vi "Graph_range_select_slider.vi"() -> ()   [LabVIEW 2018]
panel:
  in  "X_Slider":cluster{"Slider":dbl, "Slider":dbl}(slide)={"Slider"=0.0, "Slider"=3.61890694239291} scale=3643617600.0..3643691204.0 scale format="%<%H:%M:%S\n%d/%m/%y>T"
  in  "Y_Slide":cluster{"Slider":dbl, "Slider":dbl}(slide)={"Slider"=0.0, "Slider"=6.141304347826087} scale=-0.5..2.0
  out "Graph 2":T1(graph)
  in  "Graph 1":T1(graph)=[{"Time_Stamp"=array[63091 elements], "Current_Out"=array[63091 elements]}, {"Time_Stamp"=array[63091 elements], "Current_Out"=array[63091 elements]}, {"Time_Stamp"=array[63091 elements], "Current_Out"=array[63091 elements]}, {"Time_Stamp"=array[63091 elements], "Current_Out"=array[63091 elements]}, {"Time_Stamp"=array[63091 elements], "Current_Out"=array[63091 elements]}, {"Time_Stamp"=array[63091 elements], "Current_Out"=array[63091 elements]}, {"Time_Stamp"=array[63091 elements], "Current_Out"=array[63091 elements]}]
  # "Current [uA]"
  # "Time"
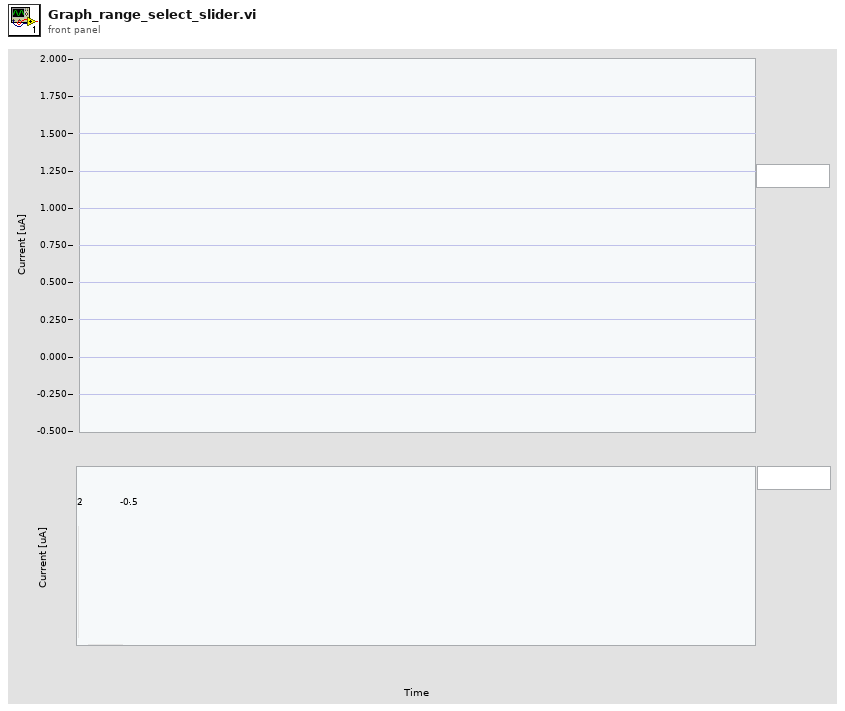
[diagram p1: front panel]
types:
  T1 = cluster{"Time_Stamp":timestamp[], "Current_Out":dbl[]}[]
  T2 = cluster{"YScale.Minimum":dbl, "YScale.Maximum":dbl}
  T3 = cluster{"XScale.Minimum":dbl, "XScale.Maximum":dbl}
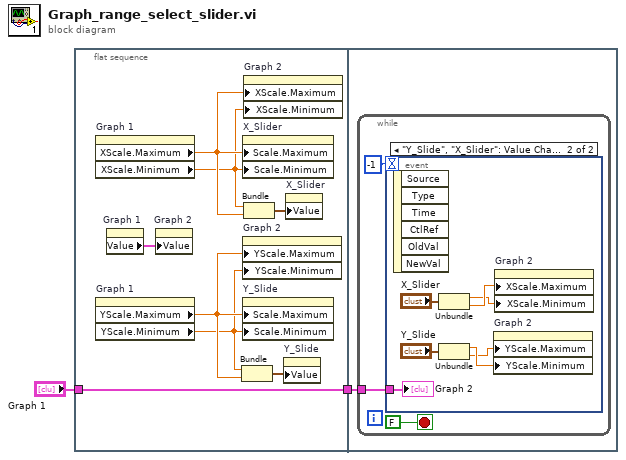
[diagram p0: block diagram]
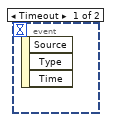
[diagram p2: hidden frame]
diagram:
  n1 = flat-sequence {
    tunnel: [w8] -> w2
    tunnel: "Graph 1" -> [w8]
    tunnel: w2 -> [w11]
    frame #0 {
      n2 = property on="Graph 1" class="XYGraph (strict)"() -> ("XScale.Maximum"=w6:dbl, "XScale.Minimum"=w5:dbl)  [unwired: 2 in, 2 out]
      n3 = property on="Graph 1" class="XYGraph (strict)"() -> ("YScale.Maximum"=w4:dbl, "YScale.Minimum"=w3:dbl)  [unwired: 2 in, 2 out]
      n4 = property on="Graph 1" class="XYGraph (strict)"() -> ("Value"=w7:T1)  [unwired: 2 in, 2 out]
      n5 = property on="Graph 2" class="XYGraph (strict)"("Value"=w7) -> ()  [unwired: 2 in, 2 out]
      n6 = Bundle("YScale.Minimum"=w3, "YScale.Maximum"=w4) -> (w9:T2)  [unwired: 1 in]
      n7 = property on="X_Slider" class="Slide (strict)"("Scale.Maximum"=w6, "Scale.Minimum"=w5) -> ()  [unwired: 2 in, 2 out]
      n8 = property on="Graph 2" class="XYGraph (strict)"("YScale.Maximum"=w4, "YScale.Minimum"=w3) -> ()  [unwired: 2 in, 2 out]
      n9 = property on="Y_Slide" class="Slide (strict)"("Scale.Maximum"=w4, "Scale.Minimum"=w3) -> ()  [unwired: 2 in, 2 out]
      n10 = property on="Graph 2" class="XYGraph (strict)"("XScale.Maximum"=w6, "XScale.Minimum"=w5) -> ()  [unwired: 2 in, 2 out]
      n11 = Bundle("XScale.Minimum"=w5, "XScale.Maximum"=w6) -> (w10:T3)  [unwired: 1 in]
      n12 = property on="Y_Slide" class="Slide (strict)"("Value"=w9) -> ()  [unwired: 2 in, 2 out]
      n13 = property on="X_Slider" class="Slide (strict)"("Value"=w10) -> ()  [unwired: 2 in, 2 out]
    }
    frame #1 {
      n14 = while {
        tunnel: w11 -> [w12]
        stop <- FALSE stop-if-true
        n15 = event shown="[1] \"Y_Slide\", \"X_Slider\": Value Change" {
          selector: _ -> [_ _]
          dyn-events: _ -> [_ _]
          timeout: -1 -> [_ _]
          tunnel: w12 -> [_ w15]
          event Timeout {
            n16 = event-data() -> ()  [unwired: 1 in, 3 out]
          }
          event "Y_Slide", "X_Slider": Value Change {
            n17 = event-data() -> ()  [unwired: 1 in, 6 out]
            n18 = Unbundle("X_Slider") -> ("Slider"=w16:dbl, "Slider"=w17:dbl)
            n19 = Unbundle("Y_Slide") -> ("Slider"=w20:dbl, "Slider"=w19:dbl)
            n20 = property on="Graph 2" class="XYGraph (strict)"("YScale.Maximum"=w19, "YScale.Minimum"=w20) -> ()  [unwired: 2 in, 2 out]
            n21 = property on="Graph 2" class="XYGraph (strict)"("XScale.Maximum"=w17, "XScale.Minimum"=w16) -> ()  [unwired: 2 in, 2 out]
            "Graph 2" <- w15
          }
        }
      }
    }
  }
